vi "variant_4d.vi"(3 "variant":variant) -> (1 "data":dbl[][][][](array[numeric]))   [LabVIEW 2014]
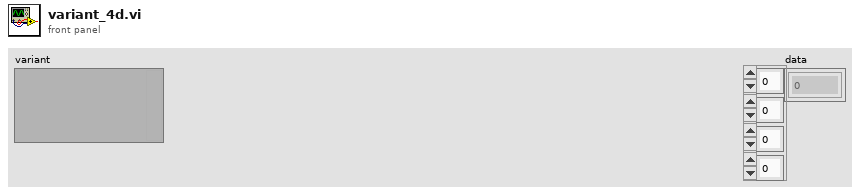
[diagram p1: front panel]
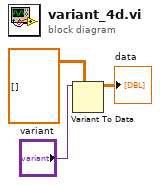
[diagram p0: block diagram]
diagram:
  n1 = Variant To Data(type=dbl[][][][] [], Variant="variant") -> (data=→"data":dbl[][][][])  [unwired: 1 in, 1 out]
